vi "GetDstTo1stPt.vi"(8 "error in (no error)":errorcluster, 11 "CarexData in":refnum<class "ExpData.lvclass">) -> (0 "error out":errorcluster, 1 "Dst to 1st Pt":dbl[](graph), 2 "Time":dbl[](array[numeric]), 3 "CarexData Out":refnum<class "ExpData.lvclass">)   [LabVIEW 2014, in "ExpData.lvclass"]
uses:
  ExpData.lvclass
  <vilib>/Analysis/NI_AALPro.lvlib
  <vilib>/Analysis/5stat.llb/RMS (DBL).vi
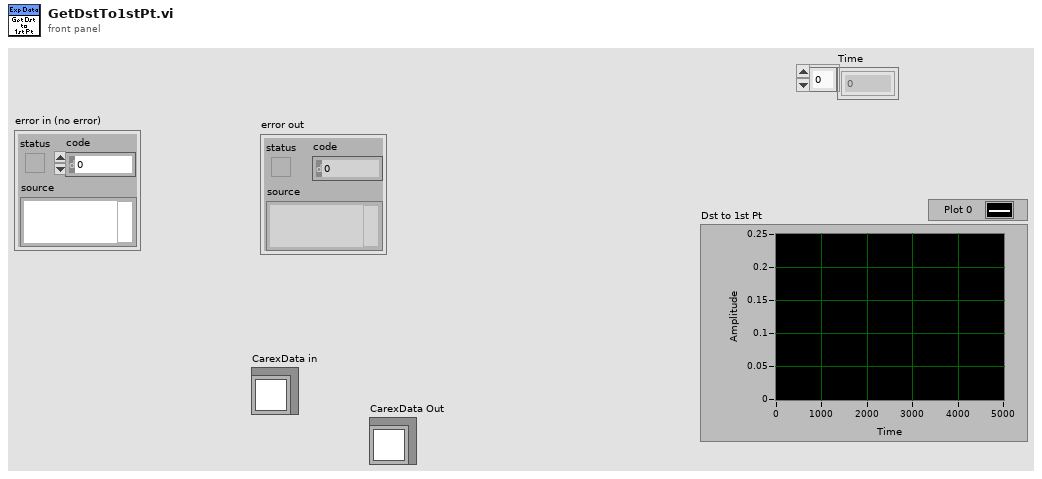
[diagram p1: front panel]
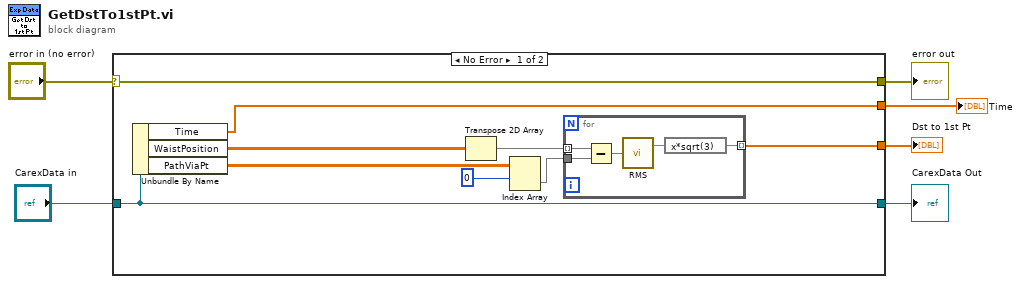
[diagram p0: block diagram]
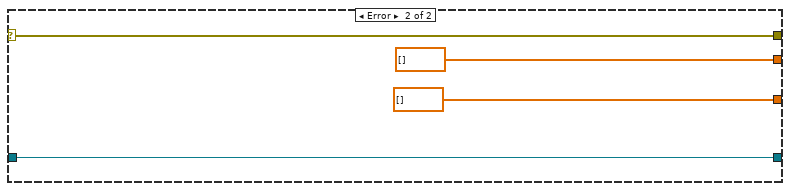
[diagram p2: hidden frame]
diagram:
  n1 = case shown="No Error" "error in (no error)" {
    selector: "error in (no error)" -> [w10 w24]
    tunnel: [w10 w24] -> w6
    tunnel: "CarexData in" -> [w11 w23]
    tunnel: [w11 w23] -> w3
    tunnel: [w7 dbl[] []] -> w2
    tunnel: [w8 dbl[] [] ("Time")] -> w1
    frame No Error {
      n2 = Unbundle By Name(w11) -> ("Time"=w8:dbl[], "WaistPosition"=w13:dbl[][], "PathViaPt"=w15:dbl[][])
      n3 = Transpose 2D Array(2D array=w13) -> (transposed array=w9:dbl[][])
      n4 = Index Array(array=w15, index (row)=0) -> (element=w12:dbl[])  [unwired: 1 in]
      n5 = for {
        tunnel: w9 -> [w20] mode=indexing
        tunnel: w12 -> [w19]
        tunnel: [w16] -> w7 mode=indexing
        n6 = Subtract(x=w20, y=w19) -> (x-y=w18:dbl[])
        n7 = call-poly <vilib>:"RMS.vi"("X"=w18) -> ("rms value"=w17:dbl)  [unwired: 1 out]
        n8 = expression code="x*sqrt(3)"(w17) -> (w16:dbl)
      }
    }
    frame Error {
    }
  }
  "error out" <- w6
  "CarexData Out" <- w3
  "Dst to 1st Pt" <- w2
  "Time" <- w1
